vi "ComboBoxOpcionestxt.vi"(10 "dispositivo":string) -> (2 "array w/ subset deleted":string[](array[string]))   [LabVIEW 2016]
uses:
  <vilib>/Utility/file.llb/Read Delimited Spreadsheet (string).vi
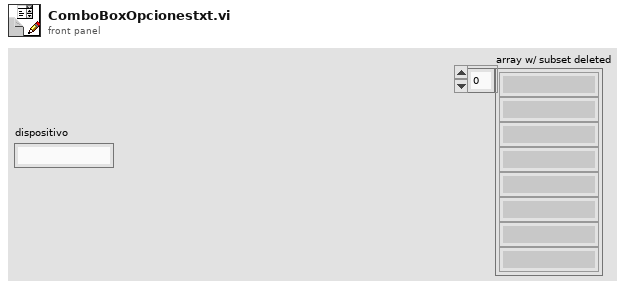
[diagram p1: front panel]
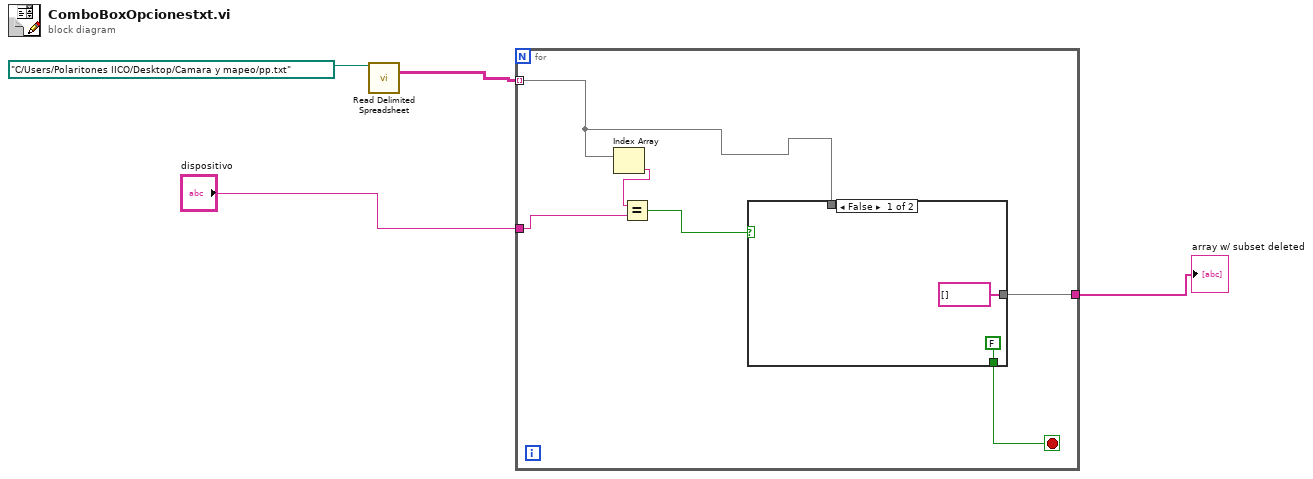
[diagram p0: block diagram]
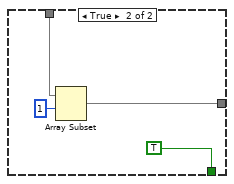
[diagram p2: hidden frame]
diagram:
  n1 = call-poly <vilib>:"Read Delimited Spreadsheet.vi"("file path (dialog if empty)"=path "C:/Users/Polaritones IICO/Desktop/Camara y mapeo/pp.txt") -> ("all rows"=w3:string[][])  [unwired: 9 in, 5 out]
  n2 = for {
    tunnel: w3 -> [w7] mode=indexing
    tunnel: "dispositivo" -> [w9]
    tunnel: [w6] -> w1
    stop <- w5 stop-if-true
    n3 = Index Array(array=w7) -> (element=w10:string)  [unwired: 1 in]
    n4 = Equal?(x=w10, y=w9) -> (x = y?=w8:bool)
    n5 = case shown="False" w8 {
      tunnel: w7 -> [_ w15]
      tunnel: [string[] [] w14] -> w6
      tunnel: [FALSE TRUE] -> w5
      frame False {
      }
      frame True {
        n6 = Array Subset(array=w15, index=1) -> (w14:string[])  [unwired: 1 in]
      }
    }
  }
  "array w/ subset deleted" <- w1
